vi "Set zero pressure to current pressure.vi"(8 "error in (no error)":errorcluster, 11 "Pressure Control in":refnum<class "Pressure Control.lvclass">) -> (0 "error out":errorcluster, 2 "New zero pressure level":dbl, 3 "Pressure Control out":refnum<class "Pressure Control.lvclass">)   [LabVIEW 2011, in "Pressure Control.lvclass"]
uses:
  Pressure Control.lvclass
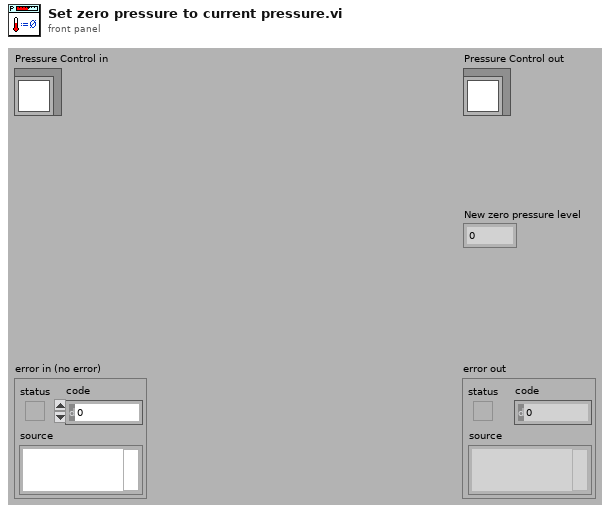
[diagram p1: front panel]
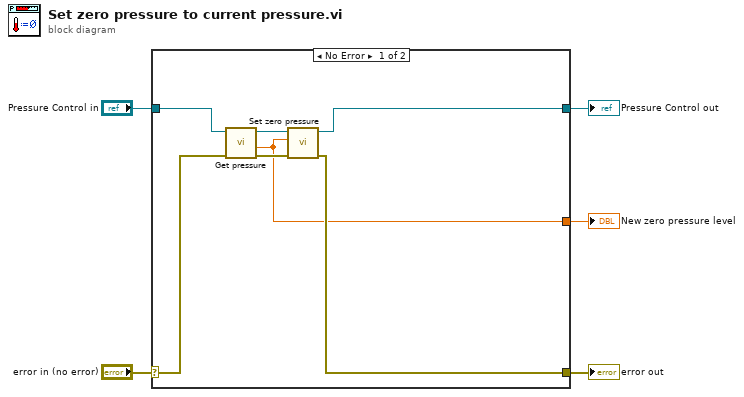
[diagram p0: block diagram]
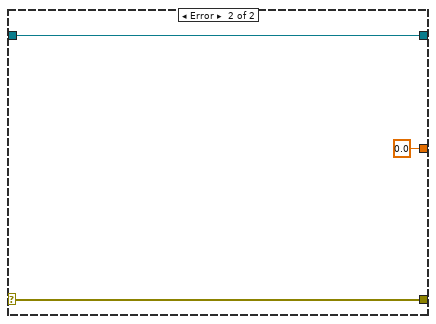
[diagram p2: hidden frame]
diagram:
  n1 = case shown="No Error" "error in (no error)" {
    selector: "error in (no error)" -> [w10 w15]
    tunnel: [w12 w15] -> w4
    tunnel: [w6 w14] -> w2
    tunnel: "Pressure Control in" -> [w7 w14]
    tunnel: [w8 0.0 ("Pressure")] -> w1
    frame No Error {
      n2 = call "Get pressure.vi"("error in (no error)"=w10, "Pressure Control in"=w7) -> ("error out"=w11:errorcluster, "Uncorrected pressure"=w8:dbl, "Pressure Control out"=w9:refnum<class "Pressure Control.lvclass">)  [unwired: 6 in, 1 out]
      n3 = call "Set zero pressure.vi"("error in (no error)"=w11, "Zero pressure level"=w8, "Pressure Control in"=w9) -> ("error out"=w12:errorcluster, "Pressure Control out"=w6:refnum<class "Pressure Control.lvclass">)  [unwired: 7 in]
    }
    frame Error {
    }
  }
  "error out" <- w4
  "Pressure Control out" <- w2
  "New zero pressure level" <- w1
